vi "Lookup or Assign Name of Client Using GUID.vi"(8 "error in (no error)":errorcluster, 10 "GUID":string, 11 "ServerListener in":refnum<class "ServerListener.lvclass">) -> (0 "error out":errorcluster, 1 "Previously connected?":bool, 2 "User Visible Name":string, 3 "ServerListener out":refnum<class "ServerListener.lvclass">)   [LabVIEW 2026, in "ServerListener.lvlib" / "ServerListener.lvclass"]
doc: "Given the GUID, this method will check to see if this client has previously connected. If it has, it will return the name that was previously used. If it has not, it will assign a new one and store the GUID in a lookup table."
uses:
  ServerListener.lvclass
  ServerListener.lvclass/ServerListener.ctl
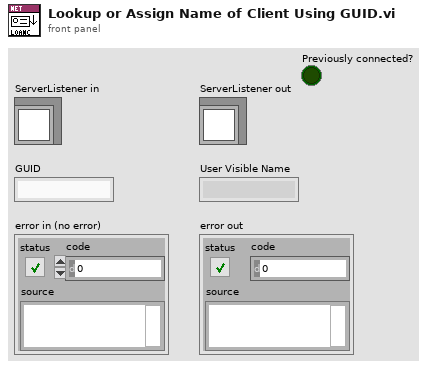
[diagram p1: front panel]
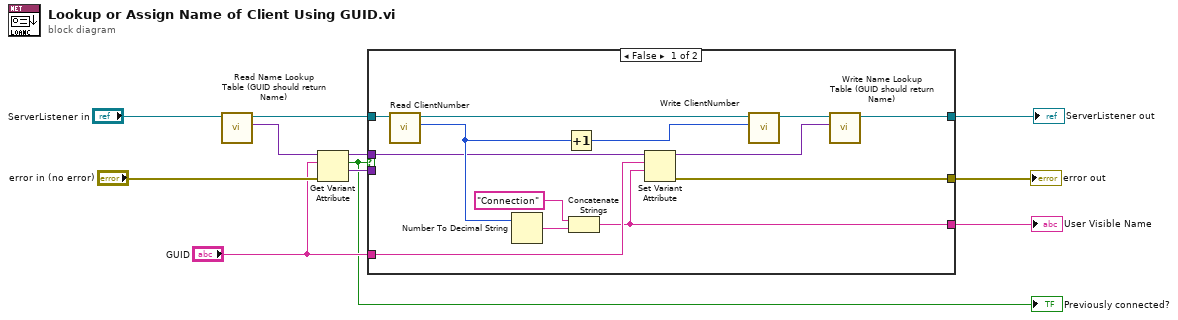
[diagram p0: block diagram]
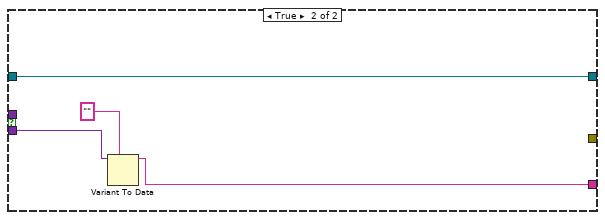
[diagram p2: hidden frame]
diagram:
  n1 = call "Read Name Lookup Table (GUID should return Name).vi"("ServerListener in"="ServerListener in") -> ("Name Lookup Table (GUID should return Name)"=w5:variant, "ServerListener out"=w4:refnum<class "ServerListener.lvclass">)  [unwired: 9 in]
  n2 = Get Variant Attribute(Variant=w5, name="GUID", error in="error in (no error)") -> (duplicate Variant=w2:variant, found=w1:bool, value=w3:variant)  [unwired: 1 in, 1 out]
  "Previously connected?" <- w1
  n3 = case shown="False" w1 {
    tunnel: w4 -> [w24 w28]
    tunnel: [w14 w28] -> w7
    tunnel: w2 -> [w18 _]
    tunnel: w3 -> [_ w27]
    tunnel: "GUID" -> [w17 _]
    tunnel: [w16 w25] -> w8
    tunnel: [w12 _] -> w11
    frame False {
      n4 = call "Read ClientNumber.vi"("ServerListener in"=w24) -> ("ClientNumber"=w20:u16, "ServerListener out"=w23:refnum<class "ServerListener.lvclass">)  [unwired: 8 in, 1 out]
      n5 = Number To Decimal String(number=w20) -> (decimal integer string=w21:string)  [unwired: 1 in]
      n6 = Increment(x=w20) -> (x+1=w19:u16)
      n7 = Concatenate Strings("Connection", w21) -> (w16:string)
      n8 = Set Variant Attribute(Variant=w18, name=w17, value=w16) -> (Variant out=w13:variant, error out=w12:errorcluster)  [unwired: 1 in, 1 out]
      n9 = call "Write ClientNumber.vi"("ClientNumber"=w19, "ServerListener in"=w23) -> ("ServerListener out"=w15:refnum<class "ServerListener.lvclass">)  [unwired: 8 in, 1 out]
      n10 = call "Write Name Lookup Table (GUID should return Name).vi"("Name Lookup Table (GUID should return Name)"=w13, "ServerListener in"=w15) -> ("ServerListener out"=w14:refnum<class "ServerListener.lvclass">)  [unwired: 9 in]
    }
    frame True {
      n11 = Variant To Data(type="", Variant=w27) -> (data=w25:string)  [unwired: 1 in, 1 out]
    }
  }
  "error out" <- w11
  "User Visible Name" <- w8
  "ServerListener out" <- w7
